vi "%Acquired.vi"(8 "error in (no error)":errorcluster, 11 "CCDCamera in":refnum<class "CCDCamera.lvclass">) -> (0 "error out":errorcluster, 3 "CCDCamera out":refnum<class "CCDCamera.lvclass">)   [LabVIEW 2018, in "CCDCamera.lvclass"]
uses:
  CCDCamera.lvclass
  Interface/Interface.lvclass
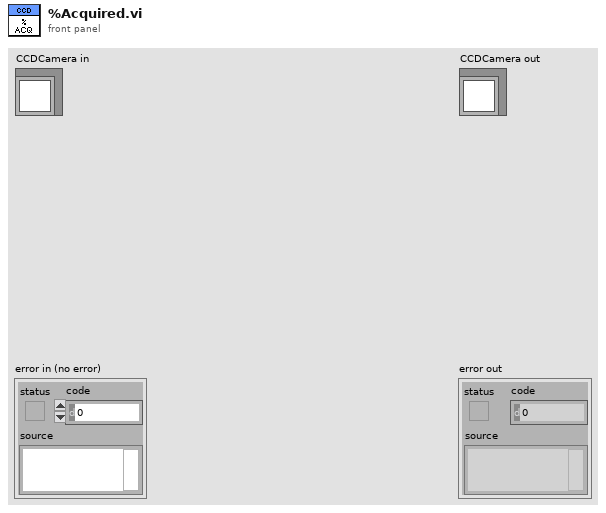
[diagram p1: front panel]
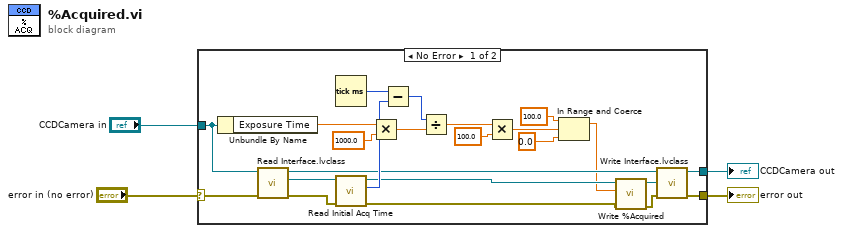
[diagram p0: block diagram]
diagram:
  n1 = case shown="No Error" "error in (no error)" {
    selector: "error in (no error)" -> [w14 w29]
    tunnel: [w11 w29] -> w2
    tunnel: [w12 w28] -> w1
    tunnel: "CCDCamera in" -> [w17 w28]
    frame No Error {
      n2 = Unbundle By Name(w17) -> ("Exposure Time"=w27:sgl)
      n3 = call-dynamic "Read Interface.lvclass.vi"("error in (no error)"=w14, "CCDCamera in"=w17) -> ("error out"=w13:errorcluster, "Interface.lvclass"=w16:refnum<class "Interface.lvclass">, "CCDCamera out"=w10:refnum<class "CCDCamera.lvclass">)  [unwired: 7 in]
      n4 = Tick Count (ms)() -> (millisecond timer value=w18:u32)
      n5 = call-dynamic "Read Initial Acq Time.vi"("error in (no error)"=w13, "Interface in"=w16) -> ("error out"=w8:errorcluster, "Initial Acq Time"=w15:u32, "Interface out"=w9:refnum<class "Interface.lvclass">)  [unwired: 7 in]
      n6 = Multiply(x=w27, y=1000.0) -> (x*y=w25:dbl)
      n7 = Subtract(x=w18, y=w15) -> (x-y=w24:u32)
      n8 = Divide(x=w24, y=w25) -> (x/y=w23:dbl)
      n9 = Multiply(x=w23, y=100.0) -> (x*y=w19:dbl)
      n10 = In Range and Coerce(upper limit=100.0 ("y"), x=w19, lower limit=0.0) -> (coerced(x)=w5:dbl)  [unwired: 1 out]
      n11 = call-dynamic "Write %Acquired.vi"("error in (no error)"=w8, "% Acquired"=w5, "Interface in"=w9) -> ("error out"=w6:errorcluster, "Interface out"=w7:refnum<class "Interface.lvclass">)  [unwired: 7 in]
      n12 = call-dynamic "Write Interface.lvclass.vi"("error in (no error)"=w6, "Interface.lvclass"=w7, "CCDCamera in"=w10) -> ("error out"=w11:errorcluster, "CCDCamera out"=w12:refnum<class "CCDCamera.lvclass">)  [unwired: 7 in]
    }
    frame Error {
    }
  }
  "error out" <- w2
  "CCDCamera out" <- w1
